vi "CLSUIP_Handle Tree Multi-Select.vi"(4 "Subpanel":refnum<vi>, 8 "error in (no error)":errorcluster, 9 "Bounds in":T1, 10 "Origin in":T2, 11 "Old VI":refnum<vi>) -> (0 "error out":errorcluster, 1 "Bounds out":T1, 2 "Origin out":T2, 3 "New VI":refnum<vi>)   [LabVIEW 2021, in "ChooseImplementation.lvlib"]
uses:
  <resource>/Framework/Providers/LVClassLibrary/ChooseImplementation/ChooseImplementation.lvlib
  <vilib>/Utility/miscctls.llb/LVRectTypeDef.ctl
  <vilib>/Utility/miscctls.llb/LVPointTypeDef.ctl
  <resource>/Framework/Providers/LVClassLibrary/ChooseImplementation/CLSUIP_Multi Select Message.vi
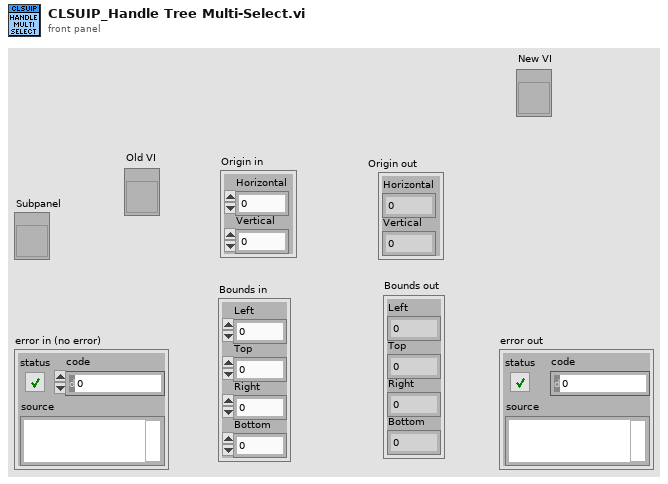
[diagram p1: front panel]
types:
  T1 = typedef "LVRectTypeDef.ctl" = cluster{"Left":i16, "Top":i16, "Right":i16, "Bottom":i16}
  T2 = typedef "LVPointTypeDef.ctl" = cluster{"Horizontal":i16, "Vertical":i16}
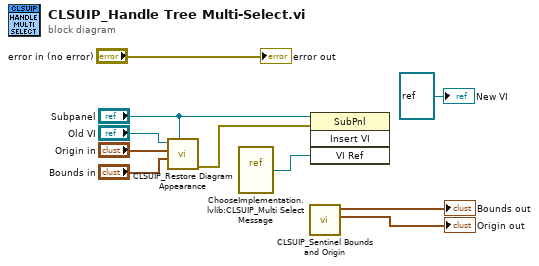
[diagram p0: block diagram]
diagram:
  n1 = call <resource>:"CLSUIP_Restore Diagram Appearance.vi"("Subpanel"="Subpanel", "Bounds"="Bounds in", "Origin"="Origin in", "Inserted VI"="Old VI") -> ("error out"=w5:errorcluster)  [unwired: 7 in]
  n2 = vi-ref "ChooseImplementation.lvlib:CLSUIP_Multi Select Message.vi"() -> (w4:refnum<vi>)
  n3 = call <resource>:"CLSUIP_Sentinel Bounds and Origin.vi"() -> ("Sentinel Origin"=→"Origin out":T2, "Sentinel Bounds"=→"Bounds out":T1)  [unwired: 10 in]
  n4 = invoke on="Invoke Node" class="SubPnl" method="Insert VI"(reference="Subpanel", error in=w5, "VI Ref"=w4) -> ()  [unwired: 1 in, 4 out]
  "New VI" <- refnum<vi> refnum ("New VI")
  "error out" <- "error in (no error)"
